vi "Single Triger.vi"(9 "Channel":string="1", 10 "VNA Model:":enum16{"E5071C", "N5230A(C)", "N5224A"}(ring)=enum."N5224A", 11 "VISA":refnum<visa-resource-name>="TCPIP0::A-N5224A-41544.local::hislip0::INSTR") -> ()   [LabVIEW 2011]
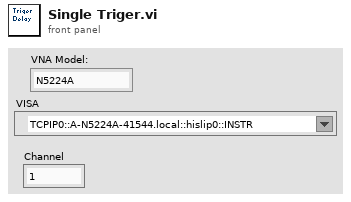
[diagram p1: front panel]
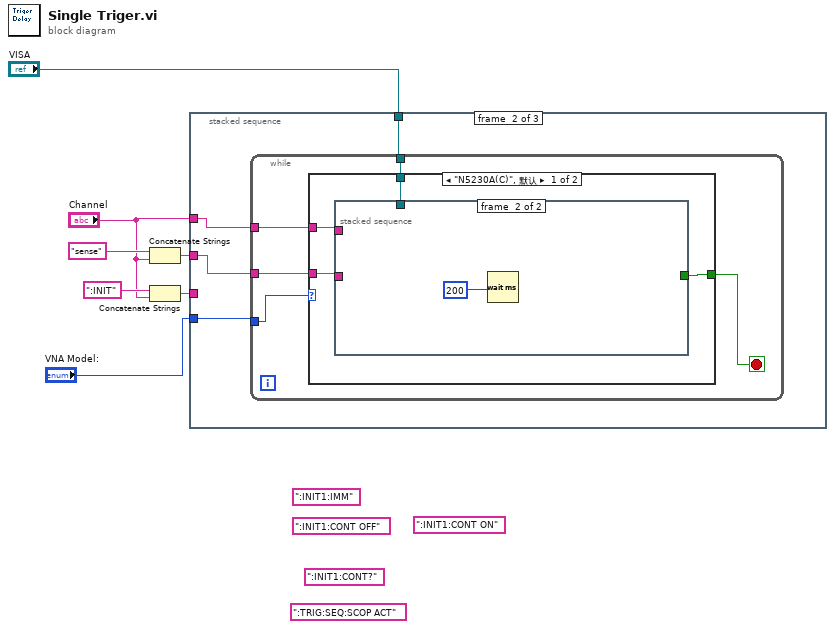
[diagram p0: block diagram]
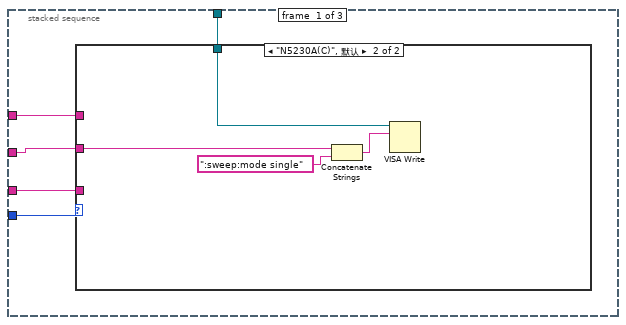
[diagram p2: hidden frame]
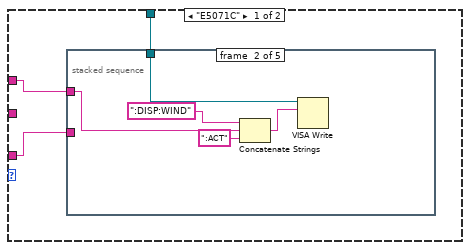
[diagram p3: hidden frame]
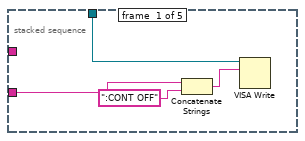
[diagram p4: hidden frame]
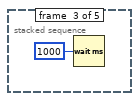
[diagram p5: hidden frame]
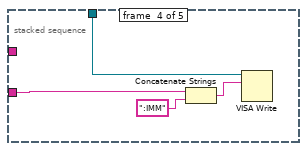
[diagram p6: hidden frame]
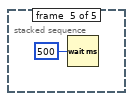
[diagram p7: hidden frame]
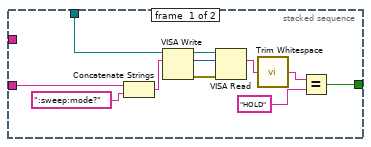
[diagram p8: hidden frame]
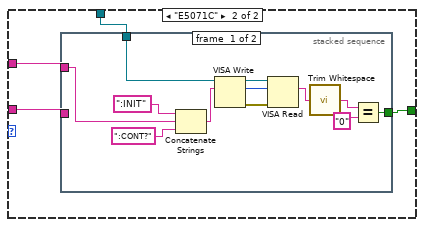
[diagram p9: hidden frame]
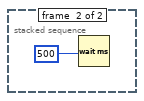
[diagram p10: hidden frame]
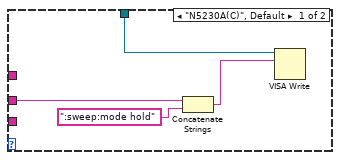
[diagram p12: hidden frame]
diagram:
  (unwired) ":TRIG:SEQ:SCOP ACT" ("write buffer")
  (unwired) ":INIT1:CONT ON" ("write buffer")
  (unwired) ":INIT1:CONT?" ("write buffer")
  (unwired) ":INIT1:CONT OFF" ("write buffer")
  (unwired) ":INIT1:IMM" ("write buffer")
  n1 = Concatenate Strings("sense" ("字符串"), "Channel") -> (w4:string)
  n2 = Concatenate Strings(":INIT" ("字符串"), "Channel") -> (w1:string)
  n3 = stacked-sequence {
    tunnel: "VISA" -> [w12 w38 w81]
    tunnel: "Channel" -> [w9 w37 w78]
    tunnel: w4 -> [w11 w36 w80]
    tunnel: "VNA Model:" -> [w10 w35 w79]
    tunnel: w1 -> [w8 _ w77]
    frame #0 {
      n4 = case shown="\"N5230A(C)\", 默认" w10 {
        tunnel: w12 -> [w15 w34]
        tunnel: w11 -> [_ w31]
        tunnel: w9 -> [w13 _]
        tunnel: w8 -> [w14 _]
        frame "E5071C" {
          n5 = stacked-sequence {
            tunnel: w15 -> [w19 w24 _ w29 _]
            tunnel: w14 -> [w18 _ _ w27 _]
            tunnel: w13 -> [_ w21 _ _ _]
            frame #0 {
              n6 = Concatenate Strings(w18, ":CONT OFF" ("write buffer")) -> (w16:string)
              n7 = VISA Write(VISA resource name=w19, write buffer=w16) -> ()  [unwired: 1 in, 3 out]
            }
            frame #1 {
              n8 = Concatenate Strings(":DISP:WIND" ("字符串"), w21, ":ACT" ("字符串")) -> (w23:string)
              n9 = VISA Write(VISA resource name=w24, write buffer=w23) -> ()  [unwired: 1 in, 3 out]
            }
            frame #2 {
              n10 = Wait (ms)(milliseconds to wait=u32 1000 ("等待时间（毫秒）")) -> ()  [unwired: 1 out]
            }
            frame #3 {
              n11 = Concatenate Strings(w27, ":IMM" ("write buffer")) -> (w26:string)
              n12 = VISA Write(VISA resource name=w29, write buffer=w26) -> ()  [unwired: 1 in, 3 out]
            }
            frame #4 {
              n13 = Wait (ms)(milliseconds to wait=u32 500 ("等待时间（毫秒）")) -> ()  [unwired: 1 out]
            }
          }
        }
        frame "N5230A(C)", Default {
          n14 = Concatenate Strings(w31, ":sweep:mode single" ("write buffer")) -> (w32:string)
          n15 = VISA Write(VISA resource name=w34, write buffer=w32) -> ()  [unwired: 1 in, 3 out]
        }
      }
    }
    frame #1 {
      n16 = while {
        tunnel: w38 -> [w43]
        tunnel: w37 -> [w41]
        tunnel: w36 -> [w40]
        tunnel: w35 -> [w39]
        stop <- w42 stop-if-true
        n17 = case shown="\"N5230A(C)\", 默认" w39 {
          tunnel: w43 -> [w47 w63]
          tunnel: [w46 w62] -> w42
          tunnel: w41 -> [w45 w61]
          tunnel: w40 -> [w44 w60]
          frame "N5230A(C)", Default {
            n18 = stacked-sequence {
              tunnel: w47 -> [w58 _]
              tunnel: [w53 _] -> w46
              tunnel: w45 -> [_ _]
              tunnel: w44 -> [w48 _]
              frame #0 {
                n19 = Concatenate Strings(w48, ":sweep:mode?" ("write buffer")) -> (w50:string)
                n20 = VISA Write(VISA resource name=w58, write buffer=w50) -> (VISA resource name out=w55:refnum<visa-resource-name>, return count=w56:u32, error out=w57:errorcluster)  [unwired: 1 in]
                n21 = VISA Read(VISA resource name=w55, byte count=w56, error in (no error)=w57) -> (read buffer=w52:string)  [unwired: 3 out]
                n22 = call <vilib>:"Trim Whitespace.vi"("string"=w52) -> ("trimmed string"=w51:string)  [unwired: 1 in]
                n23 = Equal?(x=w51, y="HOLD") -> (x = y?=w53:bool)
              }
              frame #1 {
                n24 = Wait (ms)(milliseconds to wait=u32 200 ("等待时间（毫秒）")) -> ()  [unwired: 1 out]
              }
            }
          }
          frame "E5071C" {
            n25 = stacked-sequence {
              tunnel: w63 -> [w75 _]
              tunnel: [w70 _] -> w62
              tunnel: w61 -> [w64 _]
              tunnel: w60 -> [_ _]
              frame #0 {
                n26 = Concatenate Strings(":INIT" ("write buffer"), w64, ":CONT?" ("write buffer")) -> (w67:string)
                n27 = VISA Write(VISA resource name=w75, write buffer=w67) -> (VISA resource name out=w72:refnum<visa-resource-name>, return count=w73:u32, error out=w74:errorcluster)  [unwired: 1 in]
                n28 = VISA Read(VISA resource name=w72, byte count=w73, error in (no error)=w74) -> (read buffer=w69:string)  [unwired: 3 out]
                n29 = call <vilib>:"Trim Whitespace.vi"("string"=w69) -> ("trimmed string"=w68:string)  [unwired: 1 in]
                n30 = Equal?(x=w68, y="0") -> (x = y?=w70:bool)
              }
              frame #1 {
                n31 = Wait (ms)(milliseconds to wait=u32 500 ("等待时间（毫秒）")) -> ()  [unwired: 1 out]
              }
            }
          }
        }
      }
    }
    frame #2 {
      n32 = case shown="\"E5071C\"" w79 {
        tunnel: w81 -> [w85 _]
        tunnel: w80 -> [w82 _]
        tunnel: w78 -> [_ _]
        tunnel: w77 -> [_ _]
        frame "N5230A(C)", Default {
          n33 = Concatenate Strings(w82, ":sweep:mode hold" ("write buffer")) -> (w83:string)
          n34 = VISA Write(VISA resource name=w85, write buffer=w83) -> ()  [unwired: 1 in, 3 out]
        }
        frame "E5071C" {
        }
      }
    }
  }
